vi "transitions1.vi"() -> ()   [LabVIEW 2018]
uses:
  subs/path list.vi
  <vilib>/Analysis/NI_AALPro.lvlib
panel:
  out "B":dbl=22.2 format="%.2f"
  in  "multiply factor":dbl=1000000.0 format="%.2e"
  in  "n norm":u8=5
  in  "adjustment":dbl=1.0 format="%.3f"
  in  "R_offset start":dbl=10.0 format="%.2f"
  in  "Delta T start":dbl=1.2 format="%.2f"
  in  "T mean start":dbl=2.7 format="%.2f"
  in  "# points copy":dbl=1023.0 format="%.2f"
  in  "T max":dbl=20.0 format="%.2f"
  in  "T min":dbl format="%.2f"
  in  "# points":u32=101
  in  "B max":dbl=32.0 format="%.4f"
  in  "B min":dbl=22.0 format="%.4f"
  in  "save plots?":bool=TRUE
  in  "format":string="%.6e"
  in  "temperatures":dbl[](array[numeric])=[0.478, 0.813, 1.165, 1.47, 1.82, 2.1, 2.5, 3.0, 3.5, 4.2, 5.0, 6.0, 7.0, 8.0, 9.0, 10.0, 11.0] format="%.4f"
  out "plotted data":cluster{dbl[], dbl[]}[](graph)
  in  "type of interpolation":u16(ring) items=["linear", "cubic spline", "polynomial"]
  in  "y domain":u16(ring) items=["channel A"]
  in  "x domain":u16(ring) items=["B (rising field)", "B (falling field)"]
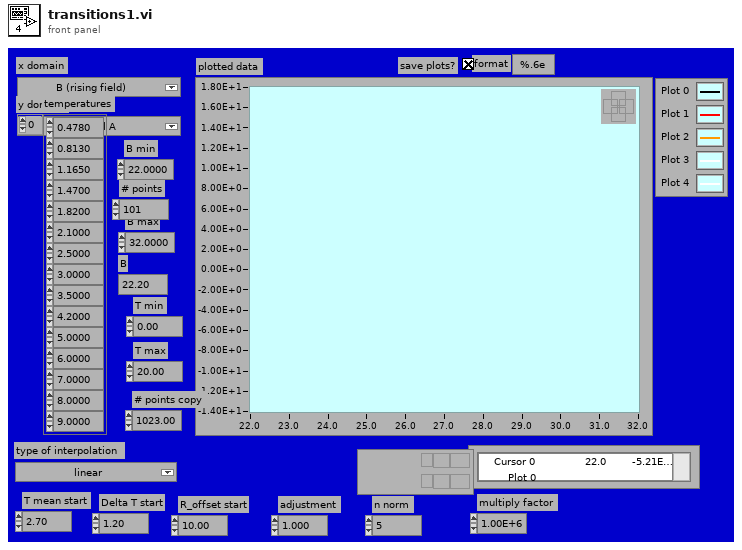
[diagram p1: front panel]
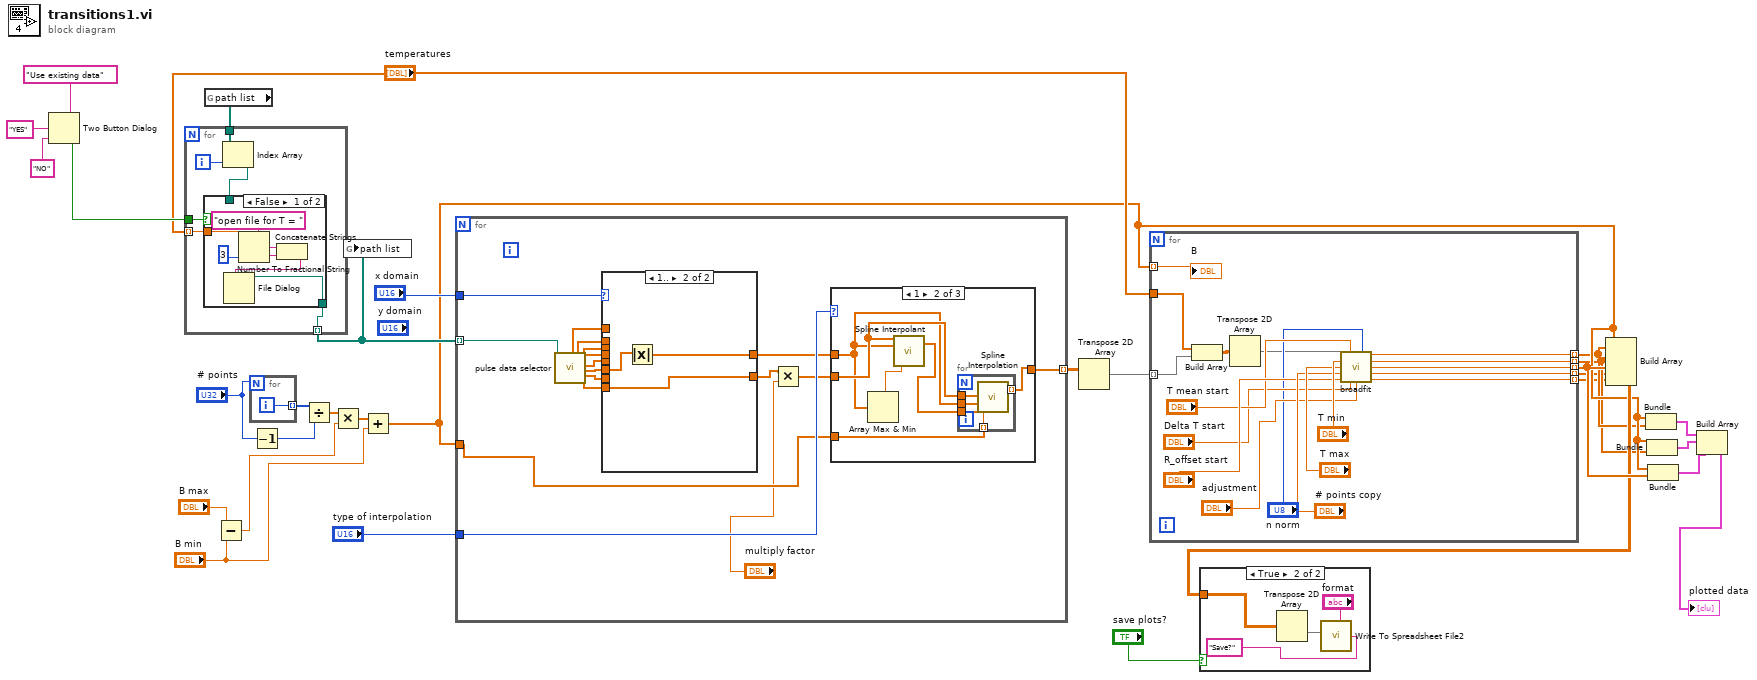
[diagram p0: block diagram]
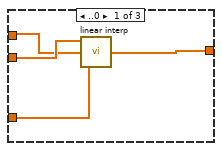
[diagram p4: hidden frame]
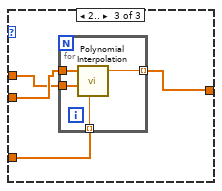
[diagram p5: hidden frame]
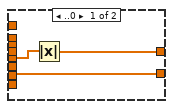
[diagram p6: hidden frame]
diagram:
  n1 = Two Button Dialog(message="Use existing data", 1:"NO", 2:"YES") -> (T button?=w24:bool)
  n2 = global read "path list.vi" "path list"() -> (w28:path[])
  n3 = for {
    tunnel: "temperatures" -> [w37] mode=indexing
    tunnel: [w36] -> w29 mode=indexing
    tunnel: w28 -> [w34]
    tunnel: w24 -> [w35]
    i -> [w33]
    n4 = Index Array(array=w34, index=w33) -> (element=w32:path)
    n5 = case shown="False" w35 {
      tunnel: w37 -> [w39 _]
      tunnel: [w38 w44] -> w36
      tunnel: w32 -> [_ w44]
      frame False {
        n6 = Number To Fractional String(number=w39, precision (6)=3) -> (F-format string=w42:string)  [unwired: 2 in]
        n7 = Concatenate Strings("open file for T = ", w42) -> (w43:string)
        n8 = File Dialog(7:w43) -> (3:w38:path)  [unwired: 6 in, 3 out]
      }
      frame True {
      }
    }
  }
  n9 = Subtract(x="B max", y="B min") -> (x-y=w18:dbl)
  n10 = for {
    N: "# points" -> [_]
    tunnel: [w45] -> w20 mode=indexing
    i -> [w45]
  }
  n11 = Decrement(x="# points") -> (x-1=w21:u32)
  n12 = Divide(x=w20, y=w21) -> (x/y=w17:dbl[])
  n13 = Multiply(x=w17, y=w18) -> (x*y=w16:dbl[])
  n14 = global write "path list.vi" "path list"(w29) -> ()
  n15 = Add(x=w16, y="B min") -> (x+y=w9:dbl[])
  n16 = for {
    tunnel: "x domain" -> [w54]
    tunnel: "type of interpolation" -> [w52]
    tunnel: w29 -> [w53] mode=indexing
    tunnel: w9 -> [w50]
    tunnel: [w49] -> w14 mode=indexing
    n17 = call "pulse data selector.vi"("file path (dialog if empty)"=w53) -> ("time rising"=w57:dbl[], "time falling"=w58:dbl[], "dB/dt rising"=w56:dbl[], "dB/dt falling"=w55:dbl[], "B rising"=w61:dbl[], "B falling"=w62:dbl[], "ch A rising"=w59:dbl[], "ch A falling"=w60:dbl[])  [unwired: 6 in, 5 out]
    n18 = case shown="1.." w54 {
      tunnel: w57 -> [_ _]
      tunnel: w58 -> [_ _]
      tunnel: w59 -> [w87 _]
      tunnel: w60 -> [_ w89]
      tunnel: w61 -> [w88 _]
      tunnel: w62 -> [_ w91]
      tunnel: w56 -> [_ _]
      tunnel: w55 -> [_ _]
      tunnel: [w87 w89] -> w48
      tunnel: [w86 w90] -> w51
      frame ..0 {
        n19 = Absolute Value(x=w88) -> (abs(x)=w86:dbl[])
      }
      frame 1.. {
        n20 = Absolute Value(x=w91) -> (abs(x)=w90:dbl[])
      }
    }
    n21 = Multiply(x=w48, y="multiply factor") -> (x*y=w47:dbl[])
    n22 = case shown="1" w52 {
      tunnel: w51 -> [w65 w69 w80]
      tunnel: w47 -> [w66 w70 w81]
      tunnel: [w63 w67 w78] -> w49
      tunnel: w50 -> [w64 w71 w79]
      frame ..0 {
        n23 = call "linear interp.vi"("x array"=w64, "X data"=w65, "Y data"=w66) -> ("y"=w63:dbl[])
      }
      frame 1 {
        n24 = Array Max & Min(array=w69) -> (max value=w72:dbl)  [unwired: 3 out]
        n25 = call <vilib>:"Spline Interpolant.vi"("final boundary"=w72, "X"=w69, "Y"=w70) -> ("Interpolant"=w68:dbl[])  [unwired: 1 in, 1 out]
        n26 = for {
          tunnel: w71 -> [w77] mode=indexing
          tunnel: w70 -> [w76]
          tunnel: w69 -> [w75]
          tunnel: w68 -> [w74]
          tunnel: [w73] -> w67 mode=indexing
          n27 = call <vilib>:"Spline Interpolation.vi"("x value"=w77, "Interpolant"=w74, "X"=w75, "Y"=w76) -> ("interpolation value"=w73:dbl)  [unwired: 1 out]
        }
      }
      frame 2.. {
        n28 = for {
          tunnel: w81 -> [w85]
          tunnel: w80 -> [w84]
          tunnel: w79 -> [w83] mode=indexing
          tunnel: [w82] -> w78 mode=indexing
          n29 = call <vilib>:"Polynomial Interpolation.vi"("x value"=w83, "X"=w84, "Y"=w85) -> ("interpolation value"=w82:dbl)  [unwired: 2 out]
        }
      }
    }
  }
  n30 = Transpose 2D Array(2D array=w14) -> (transposed array=w13:dbl[][])
  n31 = for {
    tunnel: w9 -> [w94] mode=indexing
    tunnel: "temperatures" -> [w109]
    tunnel: w13 -> [w108] mode=indexing
    tunnel: [w98] -> w8 mode=indexing
    tunnel: [w97] -> w7 mode=indexing
    tunnel: [w96] -> w11 mode=indexing
    tunnel: [w93] -> w2 mode=indexing
    tunnel: [w92] -> w1 mode=indexing
    n32 = Build Array(w109, w108) -> (w107:dbl[][])
    n33 = Transpose 2D Array(2D array=w107) -> (transposed array=w95:dbl[][])
    n34 = call "broadfit.vi"("input"=w95, "T mean start"="T mean start", "n norm"="n norm", "T min"="T min", "T max"="T max", "# points"="# points copy", "R_offset start"="R_offset start", "Delta T start"="Delta T start", "adjustment"="adjustment") -> ("T mean final"=w98:dbl, "Delta T final"=w97:dbl, "R_offset final"=w96:dbl, "r_0"=w93:dbl, "sumsqu"=w92:dbl)  [unwired: 2 in]
    "B" <- w94
  }
  n35 = Build Array(w9, w8, w7, w11, w2, w1) -> (w10:dbl[][])
  n36 = case shown="True" "save plots?" {
    tunnel: w10 -> [_ w110]
    frame False {
    }
    frame True {
      n37 = Transpose 2D Array(2D array=w110) -> (transposed array=w112:dbl[][])
      n38 = call "Write To Spreadsheet File2.vi"("dialogue"="Save?", "format (%.3f)"="format", "2D data"=w112) -> ()  [unwired: 5 in, 1 out]
    }
  }
  n39 = Bundle(w9, w8) -> (w6:cluster{dbl[], dbl[]})  [unwired: 1 in]
  n40 = Bundle(w9, w7) -> (w5:cluster{dbl[], dbl[]})  [unwired: 1 in]
  n41 = Bundle(w9, w11) -> (w4:cluster{dbl[], dbl[]})  [unwired: 1 in]
  n42 = Build Array(w6, w5, w4) -> (→"plotted data":cluster{dbl[], dbl[]}[])
